vi "Create Group.vi"(4 "Channel Resources (Unset)":string[](array[string]), 5 "Raw Values (F)":bool, 6 "Channel Names":string[](array[string]), 7 "Group Type":refnum<class "GroupAbstract.lvclass">, 8 "error in (no error)":errorcluster, 9 "Publish Config (Local Only)":T1, 10 "Group Name":string, 11 "Task in":refnum<class "Task.lvclass">) -> (0 "error out":errorcluster, 2 "Group":refnum<class "GroupAbstract.lvclass">, 3 "Task out":refnum<class "Task.lvclass">)   [LabVIEW 2020, in "Volatus.lvlib" / "Task.lvclass"]
uses:
  Task.lvclass
  lv-vecto/Vecto/GroupAbstract/GroupAbstract.lvclass
  lv-vecto/Vecto/Publish Config.ctl
  Task.lvclass/Task.ctl
  lv-vecto/Vecto/Group Info.ctl
  TelemetryAPI/TelemetryAPI.lvclass
  lv-vecto/Vecto/Vecto.lvlib
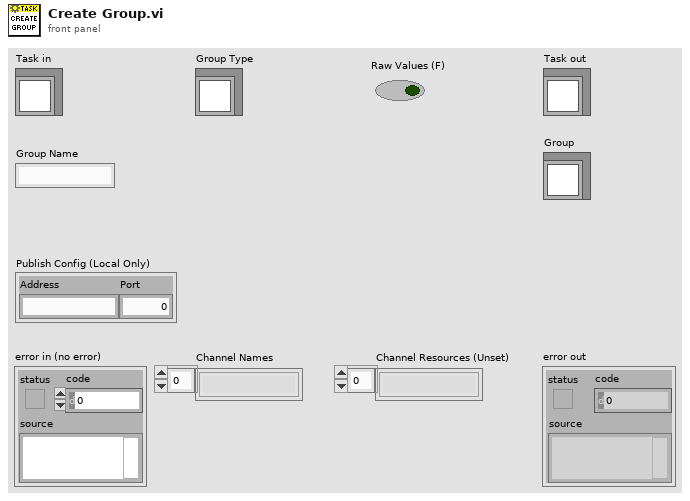
[diagram p1: front panel]
types:
  T1 = typedef "Vecto.lvlib/Publish Config.ctl" = cluster{"Address":string, "Port":u16}
  T2 = typedef "Vecto.lvlib/Group Info.ctl" = cluster{"System":string, "Cluster":string, "Node":string, "Task":string, "Name":string}
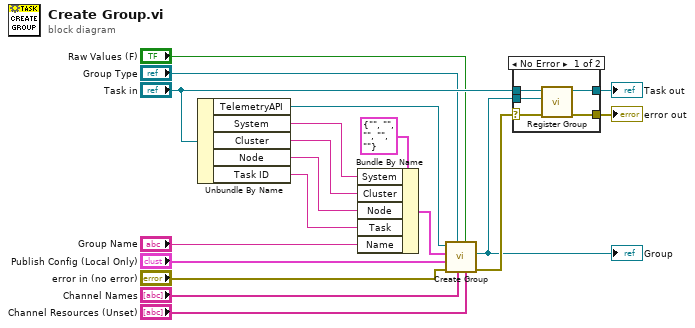
[diagram p0: block diagram]
diagram:
  n1 = Unbundle By Name("Task in") -> ("TelemetryAPI"=w17:refnum<class "TelemetryAPI.lvclass">, "System"=w4:string, "Cluster"=w5:string, "Node"=w6:string, "Task ID"=w7:string)
  n2 = Bundle By Name(cluster=T2 {"System"="", "Cluster"="", "Node"="", "Task"="", "Name"=""} ("Group Info"), "System"=w4, "Cluster"=w5, "Node"=w6, "Task"=w7, "Name"="Group Name") -> (w9:T2)
  n3 = call "Create Group.vi"("Channel Resources (Unset)"="Channel Resources (Unset)", "Raw Values (F)"="Raw Values (F)", "Channel Names"="Channel Names", "Group Type"="Group Type", "error in (no error)"="error in (no error)", "Publish Config (None)"="Publish Config (Local Only)", "Group Info"=w9, "TelemetryAPI in"=w17) -> ("error out"=w19:errorcluster, "Group"=w1:refnum<class "GroupAbstract.lvclass">)  [unwired: 1 in, 1 out]
  "Group" <- w1
  n4 = case shown="No Error" w19 {
    selector: w19 -> [w22 w25]
    tunnel: "Task in" -> [w24 w26]
    tunnel: [w23 w26] -> w3
    tunnel: [w21 w25] -> w2
    tunnel: w1 -> [w20 _]
    frame No Error {
      n5 = call "Register Group.vi"("error in (no error)"=w22, "Group"=w20, "Task in"=w24) -> ("error out"=w21:errorcluster, "Task out"=w23:refnum<class "Task.lvclass">)  [unwired: 7 in]
    }
    frame Error {
    }
  }
  "error out" <- w2
  "Task out" <- w3
